vi "User Event Init.vi"() -> (2 "Event Registration Refnum":refnum<event-registration>, 3 "user events":T1)   [LabVIEW 2021]
doc: "create user events"
uses:
  User Events.ctl
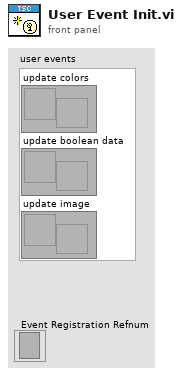
[diagram p1: front panel]
types:
  T1 = typedef "User Events.ctl" = cluster{"update colors":refnum<user-event>, "update boolean data":refnum<user-event>, "update image":refnum<user-event>}
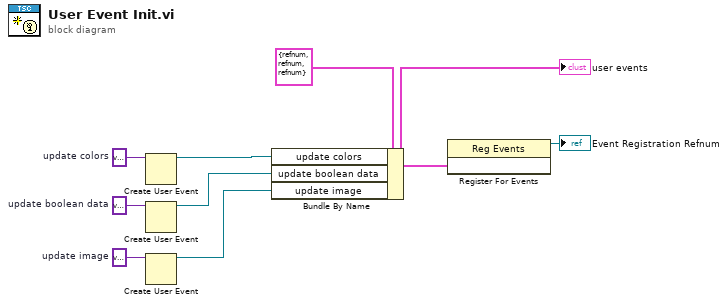
[diagram p0: block diagram]
diagram:
  w2 = variant  # update image
  w9 = variant  # update boolean data
  w8 = variant  # update colors
  n1 = Create User Event(user event datatype=w8) -> (user event=w5:refnum<user-event>)  [unwired: 1 in, 1 out]
  n2 = Create User Event(user event datatype=w9) -> (user event=w6:refnum<user-event>)  [unwired: 1 in, 1 out]
  n3 = Create User Event(user event datatype=w2) -> (user event=w1:refnum<user-event>)  [unwired: 1 in, 1 out]
  n4 = Bundle By Name(cluster=T1 {"update colors"=refnum, "update boolean data"=refnum, "update image"=refnum}, "update colors"=w5, "update boolean data"=w6, "update image"=w1) -> (w4:T1)
  "user events" <- w4
  n5 = register-events(w4) -> (reference out=→"Event Registration Refnum":refnum<event-registration>)  [unwired: 2 in, 1 out]
